vi "ClassPanel.vi"(8 "error in (no error)":errorcluster caption="entrée d'erreur (pas d'erreur)", 11 "AttoAMC.lvclass":refnum<class "AttoAMC.lvclass">) -> (0 "error out":errorcluster caption="sortie d'erreur", 3 "AttoAMC.lvclass Out":refnum<class "AttoAMC.lvclass">)   [LabVIEW 2019, in "AttoAMC.lvclass"]
uses:
  AttoAMC.lvclass
  C:/Programmes Labview/LabScanV1A/DevicesClass/BaseDevice/BaseDevice.lvclass
  AttoAMC.lvclass/AttoAMC.ctl
  BaseDevice/ClassQueueMess.ctl
  BaseDevice/Accessor/GetClassEvent.vi
panel:
  in  "FastScan":bool
  out "QuickPanRef":refnum<vi>
  in  "QuickPan":bool caption="MiseAJour"
  in  "AutoReset Ref":bool
  in  "Update Ref.":bool
  out "In Rng":bool
  in  "Target Rng":dbl=60.0 caption="Tgt. Rng.(nm)" min=1.0 step=1.0 format="%#.1f"
  out "Moving":bool
  out "ActVoltage":u32=60 caption="Act.Volt(mv)" min=1 step=1
  in  "Enable":bool
  out "Axis Model":string
  out "Valid Ref":bool
  out "BKD Lim":bool
  out "FWD Lim":bool
  in  "Axis":u8(ring) items=["1", "2", "3"]
  in  "MainProgQ":refnum<queue>
  in  "MainProgQEvent":refnum<user-event>
  out "RefPos":dbl=60.0 caption="Ref Pos(um)" min=0.1 step=0.1 format="%#.3f"
  in  "Freq.(Hz)":dbl
  in  "Ampl.(V)":dbl
  out "ActPos":dbl=60.0 caption="Actual Pos(um)" min=0.1 step=0.1 format="%#.3f"
  in  "Ctrl loop":bool
  in  "Read\nContin.":bool
  in  "Acq":bool
  in  "Stop":bool
  in  "Reset":bool caption="MiseAJour"
  in  "Target":dbl=60.0 caption="Target(um)" min=-25000.0 max=25000.0 step=0.001 format="%#.3f"
  out "Init Program":bool
  in  "Axis Name":string
  # "this MUST labeled with class name"
  # "this MUST be present and labeled \"Stop\" and \"Acq\""
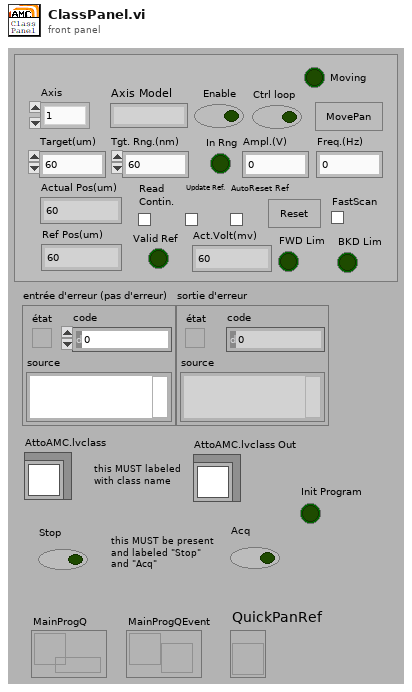
[diagram p1: front panel]
types:
  T1 = typedef "ClassQueueMess.ctl" = u16
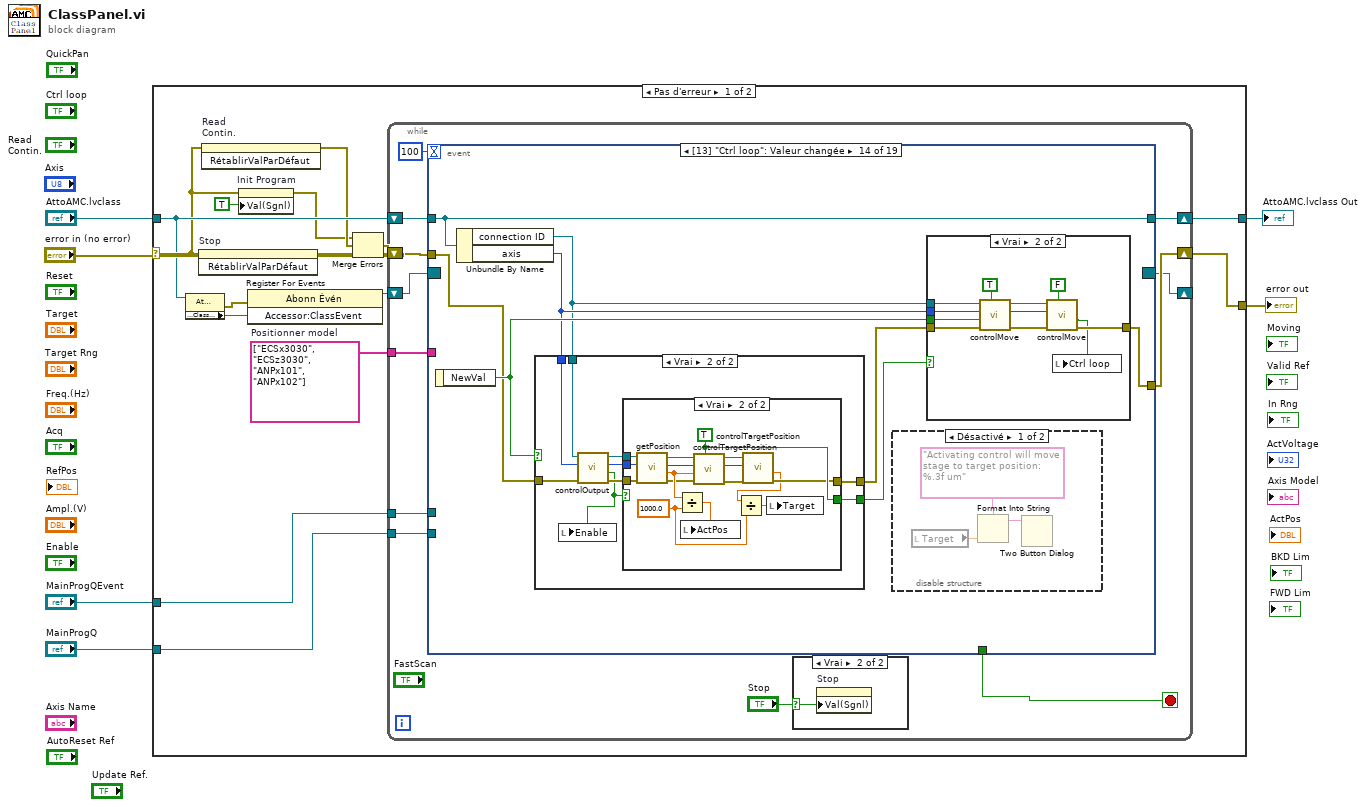
[diagram p0: block diagram]
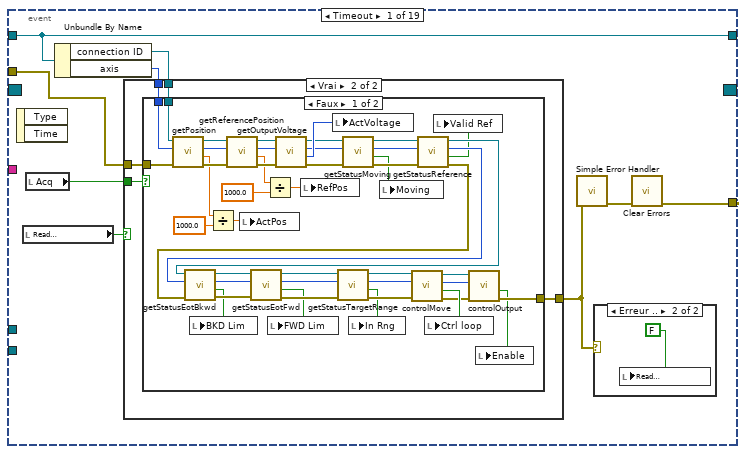
[diagram p3: hidden frame]
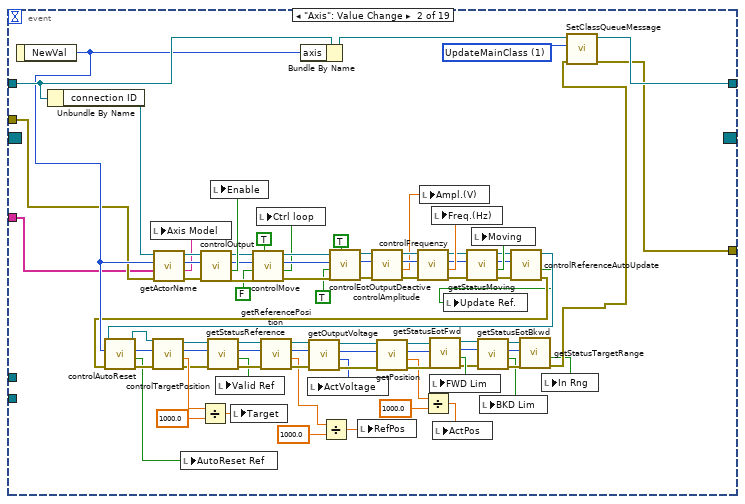
[diagram p7: hidden frame]
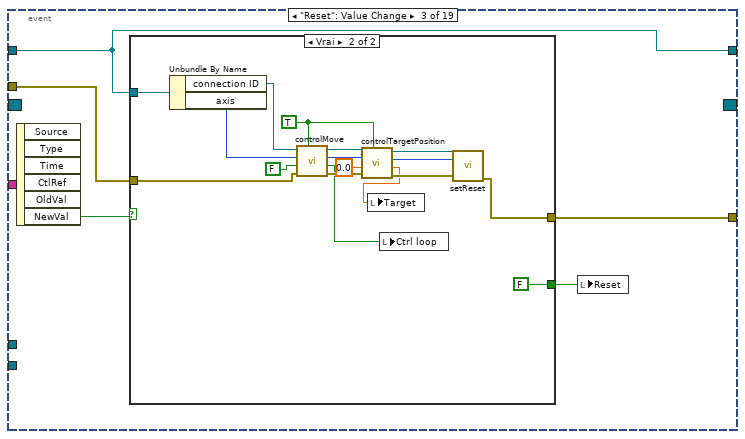
[diagram p8: hidden frame]
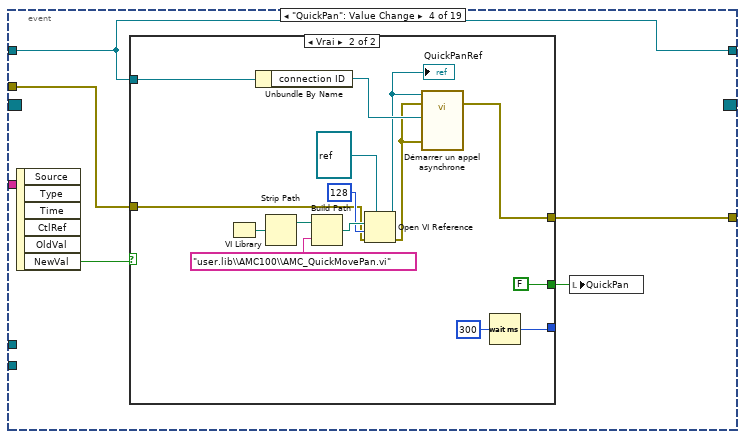
[diagram p10: hidden frame]
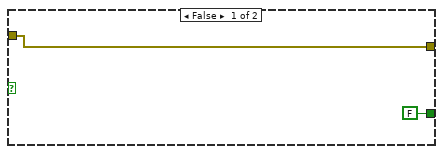
[diagram p11: hidden frame]
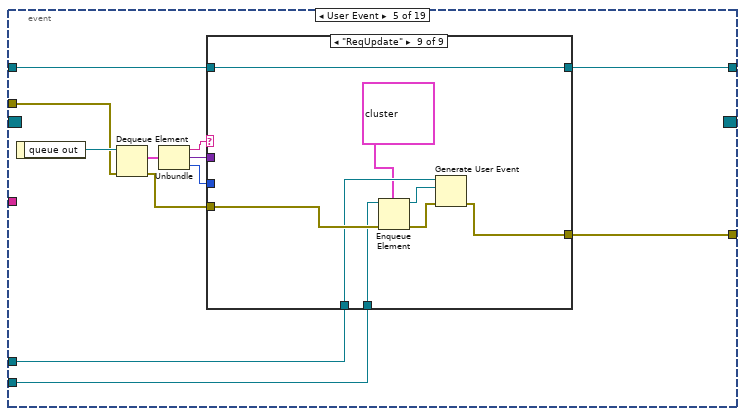
[diagram p12: hidden frame]
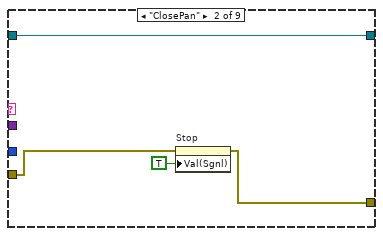
[diagram p14: hidden frame]
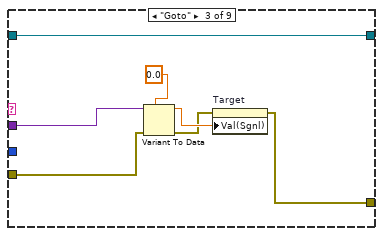
[diagram p15: hidden frame]
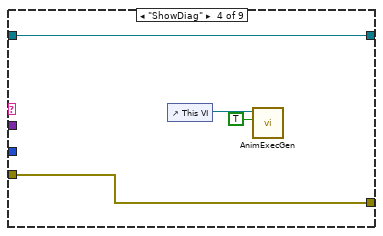
[diagram p16: hidden frame]
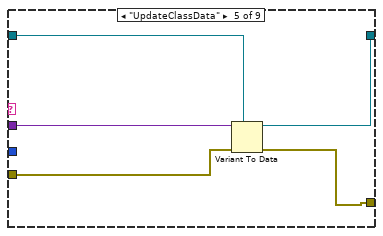
[diagram p17: hidden frame]
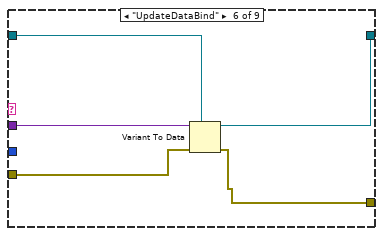
[diagram p18: hidden frame]
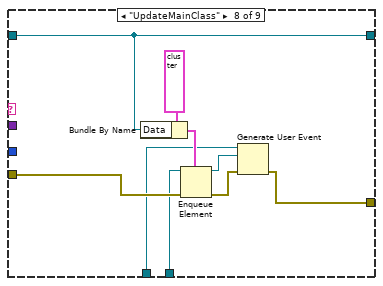
[diagram p20: hidden frame]
diagram:
  n1 = case shown="Pas d'erreur" "error in (no error)" {
    selector: "error in (no error)" -> [w8 w669]
    tunnel: [w21 w669] -> w5
    tunnel: "AttoAMC.lvclass" -> [w16 w668]
    tunnel: [w20 w668] -> w3
    tunnel: "MainProgQEvent" -> [w14 _]
    tunnel: "MainProgQ" -> [w13 _]
    frame No Error {
      w10 = string[] ["ECSx3030", "ECSz3030", "ANPx101", "ANPx102"]  # Positionner model
      n2 = property class="AttoAMC.lvclass"(reference=w16) -> (error out=w18:errorcluster, "Accessor:ClassEvent"=w17:refnum<user-event>)  [unwired: 1 in, 1 out]
      n3 = invoke on="Stop" class="Bool (strict)" method="RétablirValParDéfaut"(error in=w8) -> (error out=w19:errorcluster)  [unwired: 2 in, 2 out]
      n4 = invoke on="Read\nContin." class="Bool (strict)" method="RétablirValParDéfaut"(error in=w8) -> (error out=w11:errorcluster)  [unwired: 2 in, 2 out]
      n5 = property on="Init Program" class="Bool (strict)"(error in=w8, "Val(Sgnl)"=TRUE ("Valeur (Signalisation)")) -> (error out=w7:errorcluster)  [unwired: 1 in, 1 out]
      n6 = register-events(error in=w18, w17) -> (reference out=w15:refnum<event-registration>)  [unwired: 1 in, 1 out]
      n7 = Merge Errors(w7, w11, w19) -> (w12:errorcluster)
      n8 = while {
        shift-right: [w31] -> w21
        shift-left: w12 -> [w32]
        shift-right: [w29] -> w20
        shift-left: w16 -> [w30]
        shift-right: [w27] -> _
        shift-left: w15 -> [w28]
        tunnel: w14 -> [w26]
        tunnel: w13 -> [w25]
        tunnel: w10 -> [w24]
        stop <- w22 stop-if-true
        n9 = event shown="[13] \"Ctrl loop\": Valeur changée" {
          selector: w28 -> [_ _ _ _ _ _ _ _ _ _ _ _ _ _ _ _ _ _ _]
          dyn-events: [_ _ _ _ _ _ _ _ _ _ _ _ _ _ _ _ _ _ _] -> w27
          timeout: 100 -> [_ _ _ _ _ _ _ _ _ _ _ _ _ _ _ _ _ _ _]
          tunnel: w32 -> [w40 w172 w182 w205 w230 w290 w302 w314 w326 w338 w349 w391 w403 w414 w470 w493 w517 w615 w619]
          tunnel: [w42 w173 w181 w204 w232 w288 w301 w315 w327 w336 w348 w389 w401 w418 w466 w492 w520 _ w618] -> w31
          tunnel: w30 -> [w41 w176 w183 w206 w236 w293 w305 w322 w334 w346 w352 w399 w411 w419 w469 w490 w511 _ w620]
          tunnel: [_ _ _ _ _ _ _ _ _ _ _ _ _ _ _ w491 _ _ _] -> w22
          tunnel: [w41 w179 w183 w206 w231 w293 w305 w322 w334 w346 w352 w399 w411 w419 w468 w490 w519 _ w620] -> w29
          tunnel: w26 -> [_ _ _ _ w228 _ _ _ _ _ _ _ _ _ _ _ _ _ _]
          tunnel: w25 -> [_ _ _ _ w227 _ _ _ _ _ _ _ _ _ _ _ _ _ _]
          tunnel: w24 -> [_ w171 _ _ _ _ _ _ _ _ _ _ _ _ _ _ w518 _ _]
          event Timeout {
            n10 = event-data() -> ()  [unwired: 1 in, 2 out]
            n11 = local read "Read\nContin."() -> (w36:bool)
            n12 = local read "Acq"() -> (w37:bool)
            n13 = Unbundle By Name(w41) -> ("connection ID"=w39:refnum<k5>, "axis"=w38:u8)
            n14 = case shown="Vrai" w36 {
              tunnel: w40 -> [w45 w50]
              tunnel: [w45 w49] -> w35
              tunnel: w39 -> [_ w48]
              tunnel: w38 -> [_ w47]
              tunnel: w37 -> [_ w46]
              frame False {
              }
              frame True {
                n15 = case shown="Faux" w46 {
                  tunnel: w50 -> [w74 w96]
                  tunnel: [w54 w96] -> w49
                  tunnel: w48 -> [w73 _]
                  tunnel: w47 -> [w72 _]
                  frame False {
                    n16 = call <userlib>:"getPosition.vi"("error in"=w74, "axis in"=w72, "connection ID"=w73) -> ("error out"=w85:errorcluster, "position out"=w60:dbl, "axis out"=w94:u8, "connection ID"=w95:refnum<k5>)  [unwired: 5 in]
                    n17 = Divide(x=w60, y=1000.0) -> (x/y=w59:dbl)
                    n18 = call <userlib>:"getReferencePosition.vi"("error in"=w85, "axis in"=w94, "connection ID"=w95) -> ("error out"=w75:errorcluster, "Reference position out"=w57:dbl, "axis out"=w76:u8, "connection ID"=w77:refnum<k5>)  [unwired: 5 in]
                    n19 = local write "ActPos"(w59) -> ()
                    n20 = Divide(x=w57, y=1000.0) -> (x/y=w56:dbl)
                    n21 = call <userlib>:"getOutputVoltage.vi"("error in"=w75, "axis in"=w76, "connection ID"=w77) -> ("error out"=w70:errorcluster, "Voltage (mv)"=w71:i64, "axis out"=w68:u8, "connection ID"=w69:refnum<k5>)  [unwired: 5 in]
                    n22 = local write "RefPos"(w56) -> ()
                    n23 = local write "ActVoltage"(w71) -> ()
                    n24 = call <userlib>:"getStatusMoving.vi"("error in"=w70, "axis in"=w68, "connection ID"=w69) -> ("error out"=w84:errorcluster, "status moving out"=w67:bool, "axis out"=w92:u8, "connection ID"=w93:refnum<k5>)  [unwired: 5 in]
                    n25 = local write "Moving"(w67) -> ()
                    n26 = call <userlib>:"getStatusReference.vi"("error in"=w84, "axis in"=w92, "connection ID"=w93) -> ("error out"=w83:errorcluster, "status reference out"=w66:bool, "axis out"=w90:u8, "connection ID"=w91:refnum<k5>)  [unwired: 5 in]
                    n27 = call <userlib>:"getStatusEotBkwd.vi"("error in"=w83, "axis in"=w90, "connection ID"=w91) -> ("error out"=w82:errorcluster, "Get Stus EOT BKWD out"=w65:bool, "axis out"=w88:u8, "connection ID"=w89:refnum<k5>)  [unwired: 5 in]
                    n28 = local write "BKD Lim"(w65) -> ()
                    n29 = call <userlib>:"getStatusEotFwd.vi"("error in"=w82, "axis in"=w88, "connection ID"=w89) -> ("error out"=w81:errorcluster, "Status EOT FWD out"=w64:bool, "axis out"=w86:u8, "connection ID"=w87:refnum<k5>)  [unwired: 5 in]
                    n30 = local write "FWD Lim"(w64) -> ()
                    n31 = call <userlib>:"getStatusTargetRange.vi"("error in"=w81, "axis in"=w86, "connection ID"=w87) -> ("error out"=w78:errorcluster, "Status Target Range out"=w63:bool, "axis out"=w79:u8, "connection ID"=w80:refnum<k5>)  [unwired: 5 in]
                    n32 = local write "In Rng"(w63) -> ()
                    n33 = call <userlib>:"controlMove.vi"("error in"=w78, "axis in"=w79, "connection ID"=w80) -> ("error out"=w55:errorcluster, "controll move out"=w62:bool, "axis out"=w52:u8, "connection ID"=w51:refnum<k5>)  [unwired: 5 in]
                    n34 = local write "Ctrl loop"(w62) -> ()
                    n35 = local write "Valid Ref"(w66) -> ()
                    n36 = call <userlib>:"controlOutput.vi"("error in"=w55, "axis in"=w52, "connection ID"=w51) -> ("error out"=w54:errorcluster, "enable output out"=w53:bool)  [unwired: 5 in, 2 out]
                    n37 = local write "Enable"(w53) -> ()
                  }
                  frame True {
                  }
                }
              }
            }
            n38 = call <vilib>:"Simple Error Handler.vi"("error in (no error)"=w35) -> ("error out"=w43:errorcluster)  [unwired: 4 in, 4 out]
            n39 = case shown="Erreur .." w35 {
              frame No Error {
              }
              frame Error {
                n40 = local write "Read\nContin."(FALSE ("cas vrai")) -> ()
              }
            }
            n41 = call <vilib>:"Clear Errors.vi"("error in (no error)"=w43) -> ("error out"=w42:errorcluster)  [unwired: 5 in, 1 out]
          }
          event "Axis": Value Change {
            w178 = T1 1 items=["UpdateClassData", "UpdateMainClass"] ("Menu déroulant")
            n42 = event-data() -> ("NewVal"=w175:u8)  [unwired: 1 in]
            n43 = Unbundle By Name(w176) -> ("connection ID"=w97:refnum<k5>)
            n44 = call <userlib>:"getActorName.vi"("error in"=w172, "Actor Names"=w171, "axis in"=w175, "connection ID"=w97) -> ("error out"=w150:errorcluster, "ActorName out"=w125:string, "axis out"=w148:u8, "connection ID"=w149:refnum<k5>)  [unwired: 4 in]
            n45 = local write "Axis Model"(w125) -> ()
            n46 = call <userlib>:"controlOutput.vi"("error in"=w150, "axis in"=w148, "connection ID"=w149) -> ("error out"=w160:errorcluster, "enable output out"=w161:bool, "axis out"=w158:u8, "connection ID"=w159:refnum<k5>)  [unwired: 5 in]
            n47 = local write "Enable"(w161) -> ()
            n48 = call <userlib>:"controlMove.vi"("Set"=TRUE, "error in"=w160, "control move in"=FALSE, "axis in"=w158, "connection ID"=w159) -> ("error out"=w155:errorcluster, "controll move out"=w153:bool, "axis out"=w157:u8, "connection ID"=w156:refnum<k5>)  [unwired: 3 in]
            n49 = local write "Ctrl loop"(w153) -> ()
            n50 = Bundle By Name(cluster=w176, "axis"=w175) -> (w177:refnum<class "AttoAMC.lvclass">)
            n51 = call <userlib>:"controlEotOutputDeactive.vi"("Set"=TRUE, "error in"=w155, "enable EOT in"=TRUE, "axis in"=w157, "connection ID"=w156) -> ("error out"=w163:errorcluster, "axis out"=w162:u8, "connection ID"=w164:refnum<k5>)  [unwired: 3 in, 1 out]
            n52 = call <userlib>:"controlAmplitude.vi"("error in"=w163, "axis in"=w162, "connection ID"=w164) -> ("error out"=w168:errorcluster, "amplitude [V] out"=w166:dbl, "axis out"=w170:u8, "connection ID"=w169:refnum<k5>)  [unwired: 5 in]
            n53 = call <userlib>:"controlFrequenzy.vi"("error in"=w168, "axis in"=w170, "connection ID"=w169) -> ("error out"=w147:errorcluster, "Frequenzy [Hz] out"=w167:dbl, "axis out"=w145:u8, "connection ID"=w146:refnum<k5>)  [unwired: 5 in]
            n54 = local write "Ampl.(V)"(w166) -> ()
            n55 = local write "Freq.(Hz)"(w167) -> ()
            n56 = call <userlib>:"getStatusMoving.vi"("error in"=w147, "axis in"=w145, "connection ID"=w146) -> ("error out"=w104:errorcluster, "status moving out"=w103:bool, "axis out"=w102:u8, "connection ID"=w101:refnum<k5>)  [unwired: 5 in]
            n57 = local write "Moving"(w103) -> ()
            n58 = call <userlib>:"controlReferenceAutoUpdate.vi"("error in"=w104, "axis in"=w102, "connection ID"=w101) -> ("error out"=w100:errorcluster, "ref auto up out"=w98:bool, "connection ID"=w99:refnum<k5>)  [unwired: 5 in, 1 out]
            n59 = call <userlib>:"controlAutoReset.vi"("error in"=w100, "axis in"=w175, "connection ID"=w99) -> ("error out"=w108:errorcluster, "auto reset out"=w105:bool, "axis out"=w107:u8, "connection ID"=w106:refnum<k5>)  [unwired: 5 in]
            n60 = call <userlib>:"controlTargetPosition.vi"("error in"=w108, "axis in"=w107, "connection ID"=w106) -> ("error out"=w143:errorcluster, "Target Position out"=w144:dbl, "axis out"=w141:u8, "connection ID"=w142:refnum<k5>)  [unwired: 5 in]
            n61 = local write "AutoReset Ref"(w105) -> ()
            n62 = Divide(x=w144, y=1000.0) -> (x/y=w116:dbl)
            n63 = call <userlib>:"getStatusReference.vi"("error in"=w143, "axis in"=w141, "connection ID"=w142) -> ("error out"=w140:errorcluster, "status reference out"=w138:bool, "axis out"=w137:u8, "connection ID"=w139:refnum<k5>)  [unwired: 5 in]
            n64 = local write "Valid Ref"(w138) -> ()
            n65 = local write "Target"(w116) -> ()
            n66 = call <userlib>:"getReferencePosition.vi"("error in"=w140, "axis in"=w137, "connection ID"=w139) -> ("error out"=w136:errorcluster, "Reference position out"=w113:dbl, "axis out"=w134:u8, "connection ID"=w135:refnum<k5>)  [unwired: 5 in]
            n67 = call <userlib>:"getOutputVoltage.vi"("error in"=w136, "axis in"=w134, "connection ID"=w135) -> ("error out"=w133:errorcluster, "Voltage (mv)"=w130:i64, "axis out"=w131:u8, "connection ID"=w132:refnum<k5>)  [unwired: 5 in]
            n68 = local write "ActVoltage"(w130) -> ()
            n69 = Divide(x=w113, y=1000.0) -> (x/y=w112:dbl)
            n70 = local write "RefPos"(w112) -> ()
            n71 = call <userlib>:"getPosition.vi"("error in"=w133, "axis in"=w131, "connection ID"=w132) -> ("error out"=w128:errorcluster, "position out"=w110:dbl, "axis out"=w127:u8, "connection ID"=w129:refnum<k5>)  [unwired: 5 in]
            n72 = Divide(x=w110, y=1000.0) -> (x/y=w109:dbl)
            n73 = call <userlib>:"getStatusEotFwd.vi"("error in"=w128, "axis in"=w127, "connection ID"=w129) -> ("error out"=w124:errorcluster, "Status EOT FWD out"=w126:bool, "axis out"=w121:u8, "connection ID"=w122:refnum<k5>)  [unwired: 5 in]
            n74 = local write "FWD Lim"(w126) -> ()
            n75 = local write "ActPos"(w109) -> ()
            n76 = local write "Update Ref."(w98) -> ()
            n77 = call <userlib>:"getStatusEotBkwd.vi"("error in"=w124, "axis in"=w121, "connection ID"=w122) -> ("error out"=w123:errorcluster, "Get Stus EOT BKWD out"=w118:bool, "axis out"=w120:u8, "connection ID"=w119:refnum<k5>)  [unwired: 5 in]
            n78 = local write "BKD Lim"(w118) -> ()
            n79 = call <userlib>:"getStatusTargetRange.vi"("error in"=w123, "axis in"=w120, "connection ID"=w119) -> ("error out"=w174:errorcluster, "Status Target Range out"=w117:bool)  [unwired: 5 in, 2 out]
            n80 = local write "In Rng"(w117) -> ()
            n81 = call-dynamic "SetClassQueueMessage.vi"("ErrorIn(No Error)"=w174, "Menu déroulant"=w178, "DefaultDev.lvclass"=w177) -> ("sortie d'erreur"=w173:errorcluster, "DefaultDev.lvclass Out"=w179:refnum<class "AttoAMC.lvclass">)  [unwired: 7 in]
          }
          event "Reset": Value Change {
            n82 = event-data() -> ("NewVal"=w184:bool)  [unwired: 1 in, 5 out]
            n83 = case shown="Vrai" w184 {
              tunnel: w183 -> [_ w202]
              tunnel: w182 -> [w185 w197]
              tunnel: [w185 w201] -> w181
              tunnel: [_ FALSE] -> w180
              frame False {
              }
              frame True {
                w192 = TRUE ("Set")
                n84 = Unbundle By Name(w202) -> ("connection ID"=w199:refnum<k5>, "axis"=w198:u8)
                n85 = call <userlib>:"controlMove.vi"("Set"=w192, "error in"=w197, "control move in"=FALSE, "axis in"=w198, "connection ID"=w199) -> ("error out"=w195:errorcluster, "controll move out"=w186:bool, "axis out"=w194:u8, "connection ID"=w193:refnum<k5>)  [unwired: 3 in]
                n86 = call <userlib>:"controlTargetPosition.vi"("Set"=w192, "error in"=w195, "Target Position in"=0.0, "axis in"=w194, "connection ID"=w193) -> ("error out"=w190:errorcluster, "Target Position out"=w187:dbl, "axis out"=w188:u8, "connection ID"=w189:refnum<k5>)  [unwired: 3 in]
                n87 = local write "Target"(w187) -> ()
                n88 = local write "Ctrl loop"(w186) -> ()
                n89 = call <userlib>:"setReset.vi"("error in"=w190, "axis in"=w188, "connection ID"=w189) -> ("error out"=w201:errorcluster)  [unwired: 6 in, 2 out]
              }
            }
            n90 = local write "Reset"(w180) -> ()
          }
          event "QuickPan": Value Change {
            n91 = event-data() -> ("NewVal"=w207:bool)  [unwired: 1 in, 5 out]
            n92 = case shown="Vrai" w207 {
              tunnel: w206 -> [_ w214]
              tunnel: w205 -> [w209 w212]
              tunnel: [w209 w213] -> w204
              tunnel: [FALSE FALSE] -> w203
              tunnel: [_ w211] -> _
              frame False {
              }
              frame True {
                n93 = VI Library() -> (path=w221:path)
                n94 = Unbundle By Name(w214) -> ("connection ID"=w223:refnum<k5>)
                n95 = Strip Path(path=w221) -> (stripped path=w220:path)  [unwired: 1 out]
                n96 = Build Path(base path=w220, name or relative path="user.lib\\AMC100\\AMC_QuickMovePan.vi" ("nom ou chemin relatif")) -> (appended path=w219:path)
                n97 = Open VI Reference(type specifier VI Refnum (for type only)=refnum<vi> refnum ("spécificateur de type du refnum de VI (pour type seulement)"), vi path=w219, options=128, error in (no error)=w212) -> (vi reference=w216:refnum<vi>, error out=w217:errorcluster)  [unwired: 2 in]
                "QuickPanRef" <- w216
                n98 = call-by-ref "Démarrer un appel asynchrone"(reference=w216, error in=w217, 8:"error in (no error)"=w217, "ConnID"=w223) -> (error out=w213:errorcluster)  [unwired: 9 in, 2 out]
                n99 = Wait (ms)(milliseconds to wait=u32 300 ("attente (ms)")) -> (millisecond timer value=w211:u32)
              }
            }
            n100 = local write "QuickPan"(w203) -> ()
          }
          event User Event {
            n101 = event-data() -> ("queue out"=w234:refnum<queue>)  [unwired: 1 in]
            n102 = Dequeue Element(queue=w234, error in (no error)=w230) -> (element=w235:cluster{"Message":string, "Data":variant, i32}, error out=w229:errorcluster)  [unwired: 1 in, 2 out]
            n103 = Unbundle(w235) -> ("Message"=w226:string, "Data"=w233:variant, w225:i32)
            n104 = case shown="\"ReqUpdate\"" w226 {
              tunnel: w229 -> [w238 w241 w244 w253 w255 w260 w264 w269 w279]
              tunnel: w233 -> [_ _ w248 _ w258 w263 _ _ _]
              tunnel: w236 -> [w237 w242 w249 w252 w257 w262 w265 w270 w280]
              tunnel: [w237 w242 w249 w252 w256 w261 w265 w270 w280] -> w231
              tunnel: [w238 w240 w243 w253 w254 w259 w264 w266 w276] -> w232
              tunnel: w225 -> [_ _ _ _ _ _ _ _ _]
              tunnel: w228 -> [_ _ _ _ _ _ _ w268 w278]
              tunnel: w227 -> [_ _ _ _ _ _ _ w267 w277]
              frame Default {
              }
              frame "ClosePan" {
                n105 = property on="Stop" class="Bool (strict)"(error in=w241, "Val(Sgnl)"=TRUE ("Valeur (Signalisation)")) -> (error out=w240:errorcluster)  [unwired: 1 in, 1 out]
              }
              frame "Goto" {
                n106 = Variant To Data(error in=w244, type=0.0, Variant=w248) -> (data=w246:dbl, error out=w245:errorcluster)
                n107 = property on="Target" class="NumNb (strict)"(error in=w245, "Val(Sgnl)"=w246) -> (error out=w243:errorcluster)  [unwired: 1 in, 1 out]
              }
              frame "ShowDiag" {
                n108 = control-ref of="This VI"() -> (w251:refnum<vi>)
                n109 = call <userlib>:"AnimExecGen.vi"("Animer l'exécution ?"=TRUE, "ViRef"=w251) -> ()  [unwired: 9 in, 1 out]
              }
              frame "UpdateClassData" {
                n110 = Variant To Data(error in=w255, type=w257, Variant=w258) -> (data=w256:refnum<class "AttoAMC.lvclass">, error out=w254:errorcluster)
              }
              frame "UpdateDataBind" {
                n111 = Variant To Data(error in=w260, type=w262, Variant=w263) -> (data=w261:refnum<class "AttoAMC.lvclass">, error out=w259:errorcluster)
              }
              frame "MeasDone" {
              }
              frame "UpdateMainClass" {
                n112 = Bundle By Name(cluster=cluster{"Message":string, "Data":variant, i32} {"Message"="", "Data"=variant, 0} ("élément"), "Data"=w270) -> (w271:cluster{"Message":string, "Data":variant, i32})
                n113 = Enqueue Element(queue=w267, element=w271, error in (no error)=w269) -> (queue out=w274:refnum<queue>, error out=w273:errorcluster)  [unwired: 1 in, 1 out]
                n114 = Generate User Event(user event=w268, event data cluster=w274, error in=w273) -> (error out=w266:errorcluster)  [unwired: 1 in, 1 out]
              }
              frame "ReqUpdate" {
                n115 = Enqueue Element(queue=w277, element=cluster{"Message":string, "Data":variant, i32} {"Message"="ReqUpdate", "Data"=variant, 0} ("élément"), error in (no error)=w279) -> (queue out=w282:refnum<queue>, error out=w281:errorcluster)  [unwired: 1 in, 1 out]
                n116 = Generate User Event(user event=w278, event data cluster=w282, error in=w281) -> (error out=w276:errorcluster)  [unwired: 1 in, 1 out]
              }
            }
          }
          event "Target": Value Change {
            n117 = event-data() -> ("NewVal"=w289:dbl)  [unwired: 1 in]
            n118 = Unbundle By Name(w293) -> ("connection ID"=w292:refnum<k5>, "axis"=w291:u8)
            n119 = Multiply(x=w289, y=1000.0) -> (x*y=w287:dbl)
            n120 = call <userlib>:"controlTargetPosition.vi"("Set"=TRUE, "error in"=w290, "Target Position in"=w287, "axis in"=w291, "connection ID"=w292) -> ("error out"=w295:errorcluster, "axis out"=w296:u8, "connection ID"=w297:refnum<k5>)  [unwired: 3 in, 1 out]
            n121 = call <userlib>:"controlTargetPosition.vi"("Set"=FALSE, "error in"=w295, "axis in"=w296, "connection ID"=w297) -> ("error out"=w288:errorcluster, "Target Position out"=w284:dbl)  [unwired: 4 in, 2 out]
            n122 = Divide(x=w284, y=1000.0) -> (x/y=w283:dbl)
            n123 = local write "Target"(w283) -> ()
          }
          event "Target Rng": Value Change {
            n124 = event-data() -> ("NewVal"=w300:dbl)  [unwired: 1 in]
            n125 = Unbundle By Name(w305) -> ("connection ID"=w304:refnum<k5>, "axis"=w303:u8)
            n126 = call <userlib>:"controlTargetRange.vi"("Set"=TRUE, "error in"=w302, "Target Range in"=w300, "axis in"=w303, "connection ID"=w304) -> ("error out"=w307:errorcluster, "axis out"=w308:u8, "connection ID"=w309:refnum<k5>)  [unwired: 3 in, 1 out]
            n127 = call <userlib>:"controlTargetRange.vi"("Set"=FALSE, "error in"=w307, "axis in"=w308, "connection ID"=w309) -> ("error out"=w301:errorcluster, "Target Range out"=w299:dbl)  [unwired: 4 in, 2 out]
            n128 = local write "Target Rng"(w299) -> ()
          }
          event "Ampl.(V)": Value Change {
            n129 = event-data() -> ("NewVal"=w311:dbl)  [unwired: 1 in]
            n130 = Unbundle By Name(w322) -> ("connection ID"=w313:refnum<k5>, "axis"=w312:u8)
            n131 = call <userlib>:"controlAmplitude.vi"("Set"=TRUE, "error in"=w314, "amplitude [V] in"=w311, "axis in"=w312, "connection ID"=w313) -> ("error out"=w317:errorcluster, "axis out"=w319:u8, "connection ID"=w320:refnum<k5>)  [unwired: 3 in, 1 out]
            n132 = call <userlib>:"controlAmplitude.vi"("Set"=FALSE, "error in"=w317, "axis in"=w319, "connection ID"=w320) -> ("error out"=w315:errorcluster, "amplitude [V] out"=w316:dbl)  [unwired: 4 in, 2 out]
            n133 = local write "Ampl.(V)"(w316) -> ()
          }
          event "Freq.(Hz)": Value Change {
            n134 = event-data() -> ("NewVal"=w323:dbl)  [unwired: 1 in]
            n135 = Unbundle By Name(w334) -> ("connection ID"=w325:refnum<k5>, "axis"=w324:u8)
            n136 = call <userlib>:"controlFrequenzy.vi"("Set"=TRUE, "error in"=w326, "Frequenzy [Hz] in"=w323, "axis in"=w324, "connection ID"=w325) -> ("error out"=w329:errorcluster, "axis out"=w331:u8, "connection ID"=w332:refnum<k5>)  [unwired: 3 in, 1 out]
            n137 = call <userlib>:"controlFrequenzy.vi"("Set"=FALSE, "error in"=w329, "axis in"=w331, "connection ID"=w332) -> ("error out"=w327:errorcluster, "Frequenzy [Hz] out"=w328:dbl)  [unwired: 4 in, 2 out]
            n138 = local write "Freq.(Hz)"(w328) -> ()
          }
          event "Enable": Value Change {
            n139 = event-data() -> ("NewVal"=w337:bool)  [unwired: 1 in]
            n140 = Unbundle By Name(w346) -> ("connection ID"=w340:refnum<k5>, "axis"=w339:u8)
            n141 = call <userlib>:"controlOutput.vi"("Set"=TRUE, "error in"=w338, "enable output in"=w337, "axis in"=w339, "connection ID"=w340) -> ("error out"=w341:errorcluster, "axis out"=w342:u8, "connection ID"=w343:refnum<k5>)  [unwired: 3 in, 1 out]
            n142 = call <userlib>:"controlOutput.vi"("Set"=FALSE, "error in"=w341, "axis in"=w342, "connection ID"=w343) -> ("error out"=w336:errorcluster, "enable output out"=w335:bool)  [unwired: 4 in, 2 out]
            n143 = local write "Enable"(w335) -> ()
          }
          event "Enable": Shortcut Menu Selection (User) {
            n144 = event-data() -> ("ItemTag"=w347:string)  [unwired: 1 in, 3 out]
            n145 = Unbundle By Name(w352) -> ("connection ID"=w351:refnum<k5>, "axis"=w350:u8)
            n146 = case shown="\"Faux\", Par défaut" w347 {
              tunnel: w351 -> [_ w358 w375]
              tunnel: w350 -> [_ _ _]
              tunnel: w349 -> [w353 w357 w374]
              tunnel: [w353 w356 w373] -> w348
              frame "Faux", Default {
              }
              frame "EnableAll" {
                n147 = for {
                  N: 3 -> [_]
                  tunnel: w358 -> [w365]
                  tunnel: [w362] -> w355
                  shift-right: [w363] -> w356
                  shift-left: w357 -> [w364]
                  i -> [w360]
                  n148 = Increment(x=w360) -> (x+1=w361:i32)
                  n149 = call <userlib>:"controlOutput.vi"("Set"=TRUE, "error in"=w364, "enable output in"=TRUE, "axis in"=w361, "connection ID"=w365) -> ("error out"=w366:errorcluster, "axis out"=w367:u8, "connection ID"=w368:refnum<k5>)  [unwired: 3 in, 1 out]
                  n150 = call <userlib>:"controlOutput.vi"("Set"=FALSE, "error in"=w366, "axis in"=w367, "connection ID"=w368) -> ("error out"=w363:errorcluster, "enable output out"=w362:bool)  [unwired: 4 in, 2 out]
                }
                n151 = local write "Enable"(w355) -> ()
              }
              frame "DisableAll" {
                n152 = for {
                  N: 3 -> [_]
                  tunnel: w375 -> [w382]
                  tunnel: [w379] -> w372
                  shift-right: [w380] -> w373
                  shift-left: w374 -> [w381]
                  i -> [w377]
                  n153 = Increment(x=w377) -> (x+1=w378:i32)
                  n154 = call <userlib>:"controlOutput.vi"("Set"=TRUE, "error in"=w381, "enable output in"=FALSE, "axis in"=w378, "connection ID"=w382) -> ("error out"=w383:errorcluster, "axis out"=w384:u8, "connection ID"=w385:refnum<k5>)  [unwired: 3 in, 1 out]
                  n155 = call <userlib>:"controlOutput.vi"("Set"=FALSE, "error in"=w383, "axis in"=w384, "connection ID"=w385) -> ("error out"=w380:errorcluster, "enable output out"=w379:bool)  [unwired: 4 in, 2 out]
                }
                n156 = local write "Enable"(w372) -> ()
              }
            }
          }
          event "AutoReset Ref": Value Change {
            n157 = event-data() -> ("NewVal"=w390:bool)  [unwired: 1 in]
            n158 = Unbundle By Name(w399) -> ("connection ID"=w393:refnum<k5>, "axis"=w392:u8)
            n159 = call <userlib>:"controlAutoReset.vi"("Set"=TRUE, "error in"=w391, "auto reset in"=w390, "axis in"=w392, "connection ID"=w393) -> ("error out"=w394:errorcluster, "axis out"=w395:u8, "connection ID"=w396:refnum<k5>)  [unwired: 3 in, 1 out]
            n160 = call <userlib>:"controlAutoReset.vi"("Set"=FALSE, "error in"=w394, "axis in"=w395, "connection ID"=w396) -> ("error out"=w389:errorcluster, "auto reset out"=w388:bool)  [unwired: 4 in, 2 out]
            n161 = local write "AutoReset Ref"(w388) -> ()
          }
          event "Update Ref.": Value Change {
            n162 = event-data() -> ("NewVal"=w402:bool)  [unwired: 1 in]
            n163 = Unbundle By Name(w411) -> ("connection ID"=w405:refnum<k5>, "axis"=w404:u8)
            n164 = call <userlib>:"controlReferenceAutoUpdate.vi"("Set"=TRUE, "error in"=w403, "ref auto up in"=w402, "axis in"=w404, "connection ID"=w405) -> ("error out"=w406:errorcluster, "axis out"=w407:u8, "connection ID"=w408:refnum<k5>)  [unwired: 3 in, 1 out]
            n165 = call <userlib>:"controlReferenceAutoUpdate.vi"("Set"=FALSE, "error in"=w406, "axis in"=w407, "connection ID"=w408) -> ("error out"=w401:errorcluster, "ref auto up out"=w400:bool)  [unwired: 4 in, 2 out]
            n166 = local write "Update Ref."(w400) -> ()
          }
          event "Ctrl loop": Value Change {
            n167 = event-data() -> ("NewVal"=w417:bool)  [unwired: 1 in]
            n168 = Unbundle By Name(w419) -> ("connection ID"=w413:refnum<k5>, "axis"=w415:u8)
            n169 = case shown="Vrai" w417 {
              tunnel: [TRUE ("T button?") w426] -> w416
              tunnel: w415 -> [_ w433]
              tunnel: w414 -> [w423 w432]
              tunnel: w413 -> [_ w431]
              tunnel: [w423 w425] -> w412
              frame False {
              }
              frame True {
                n170 = call <userlib>:"controlOutput.vi"("error in"=w432, "axis in"=w433, "connection ID"=w431) -> ("error out"=w430:errorcluster, "enable output out"=w427:bool, "axis out"=w428:u8, "connection ID"=w429:refnum<k5>)  [unwired: 5 in]
                n171 = local write "Enable"(w427) -> ()
                n172 = case shown="Vrai" w427 {
                  tunnel: w430 -> [w434 w452]
                  tunnel: w429 -> [_ w451]
                  tunnel: w428 -> [_ w450]
                  tunnel: [FALSE w448] -> w426
                  tunnel: [w434 w438] -> w425
                  frame False {
                    n173 = One Button Dialog(message="Axis is not Enable!") -> ()  [unwired: 1 in, 1 out]
                  }
                  frame True {
                    w448 = TRUE ("Set")
                    w442 = 1000.0 ("y")
                    n174 = call <userlib>:"getPosition.vi"("error in"=w452, "axis in"=w450, "connection ID"=w451) -> ("error out"=w444:errorcluster, "position out"=w447:dbl, "axis out"=w445:u8, "connection ID"=w446:refnum<k5>)  [unwired: 5 in]
                    n175 = Divide(x=w447, y=w442) -> (x/y=w449:dbl)
                    n176 = local write "ActPos"(w449) -> ()
                    n177 = call <userlib>:"controlTargetPosition.vi"("Set"=w448, "error in"=w444, "Target Position in"=w447, "axis in"=w445, "connection ID"=w446) -> ("error out"=w441:errorcluster, "axis out"=w440:u8, "connection ID"=w439:refnum<k5>)  [unwired: 3 in, 1 out]
                    n178 = call <userlib>:"controlTargetPosition.vi"("error in"=w441, "axis in"=w440, "connection ID"=w439) -> ("error out"=w438:errorcluster, "Target Position out"=w437:dbl)  [unwired: 5 in, 2 out]
                    n179 = Divide(x=w437, y=w442) -> (x/y=w443:dbl)
                    n180 = local write "Target"(w443) -> ()
                  }
                }
              }
            }
            n181 = disable-structure shown="Désactivé" {
              frame Disabled {
                n182 = local read "Target"() -> (w421:dbl)
                n183 = Format Into String(format string="Activating control will move stage to target position: %.3f um" ("message"), w421) -> (resulting string=w422:string)  [unwired: 2 in, 1 out]
                n184 = Two Button Dialog(message=w422) -> ()  [unwired: 2 in, 1 out]
              }
              frame Enabled {
              }
            }
            n185 = case shown="Vrai" w416 {
              tunnel: w412 -> [w453 w460]
              tunnel: w417 -> [_ w459]
              tunnel: w415 -> [_ w458]
              tunnel: w413 -> [_ w457]
              tunnel: [w453 w456] -> w418
              frame False {
                n186 = local write "Ctrl loop"(FALSE ("Control loop")) -> ()
              }
              frame True {
                n187 = call <userlib>:"controlMove.vi"("Set"=TRUE, "error in"=w460, "control move in"=w459, "axis in"=w458, "connection ID"=w457) -> ("error out"=w461:errorcluster, "axis out"=w462:u8, "connection ID"=w465:refnum<k5>)  [unwired: 3 in, 1 out]
                n188 = call <userlib>:"controlMove.vi"("Set"=FALSE, "error in"=w461, "axis in"=w462, "connection ID"=w465) -> ("error out"=w456:errorcluster, "controll move out"=w455:bool)  [unwired: 4 in, 2 out]
                n189 = local write "Ctrl loop"(w455) -> ()
              }
            }
          }
          event "Axis Name": Shortcut Menu Selection (User) {
            n190 = event-data() -> ("ItemTag"=w467:string)  [unwired: 1 in]
            n191 = case shown="\"ChangeName\"" w467 {
              tunnel: w470 -> [w471 w480]
              tunnel: w469 -> [w472 w478]
              tunnel: [w472 w475] -> w468
              tunnel: [w471 w473] -> w466
              frame Default {
              }
              frame "ChangeName" {
                n192 = call "SaveAxisName"("Enable"=TRUE, "error in (no error)"=w480) -> ("Name"=w477:string, "Save"=w476:bool, "error out"=w474:errorcluster)  [unwired: 15 in]
                n193 = case shown="Vrai" w476 {
                  tunnel: w478 -> [w482 w489]
                  tunnel: w477 -> [_ w483]
                  tunnel: [w482 w487] -> w475
                  tunnel: w474 -> [w481 w486]
                  tunnel: [w481 w484] -> w473
                  frame False {
                  }
                  frame True {
                    w485 = T1 1 items=["UpdateClassData", "UpdateMainClass"] ("Menu déroulant")
                    n194 = Bundle By Name(cluster=w489, "AxisName"=w483) -> (w488:refnum<class "AttoAMC.lvclass">)
                    n195 = local write "Axis Name"(w483) -> ()
                    n196 = call-dynamic "SetClassQueueMessage.vi"("ErrorIn(No Error)"=w486, "Menu déroulant"=w485, "DefaultDev.lvclass"=w488) -> ("sortie d'erreur"=w484:errorcluster, "DefaultDev.lvclass Out"=w487:refnum<class "AttoAMC.lvclass">)  [unwired: 7 in]
                  }
                }
              }
            }
          }
          event "Stop": Value Change {
            n197 = event-data() -> ("NewVal"=w491:bool)  [unwired: 1 in, 5 out]
            n198 = case shown="Vrai" w491 {
              tunnel: w490 -> [_ w503]
              tunnel: w493 -> [w494 w497]
              tunnel: [w494 w496] -> w492
              frame False {
              }
              frame True {
                n199 = local read "QuickPanRef"() -> (w498:refnum<vi>)
                n200 = Unbundle By Name(w503) -> ("connection ID"=w500:refnum<k5>)
                n201 = Not A Number/Path/Refnum?(number/path/refnum=w498) -> (NaN/Path/Refnum?=w499:bool)
                n202 = case shown="Faux" w499 {
                  tunnel: w498 -> [w508 _]
                  tunnel: w497 -> [w507 w509]
                  tunnel: [w505 w509] -> w495
                  frame False {
                    n203 = invoke class="Type d'interface de VI 0" method="ValCmde.Déf"(reference=w508, error in=w507, "Control Name"="Quit" ("Nom de la commande"), "Value"=TRUE) -> (error out=w505:errorcluster)  [unwired: 1 in, 4 out]
                  }
                  frame True {
                  }
                }
                n204 = call <userlib>:"AMC_OpenCloseConn.vi"("Open"=FALSE, "error in"=w497, "ConnID"=w500) -> ("error out"=w502:errorcluster)  [unwired: 7 in, 1 out]
                n205 = Merge Errors(w502, w495) -> (w496:errorcluster)
              }
            }
          }
          event "Init Program": Value Change {
            n206 = event-data() -> ()  [unwired: 1 in, 1 out]
            n207 = Unbundle By Name(w511) -> ("axis"=w514:u8, "AxisName"=w513:string)
            n208 = property class="AttoAMC.lvclass"(reference=w511) -> ("Accessor:VisaRes"=w510:refnum<visa-resource-name>)  [unwired: 1 in, 2 out]
            n209 = call <userlib>:"AMC_OpenCloseConn.vi"("Open"=TRUE, "error in"=w517, "deviceAddress"=w510) -> ("error out"=w512:errorcluster, "connection ID"=w516:refnum<k5>)  [unwired: 7 in]
            n210 = case shown="Pas d'erreur" w512 {
              selector: w512 -> [w521 w612]
              tunnel: [w579 w608] -> w520
              tunnel: w511 -> [w602 w613]
              tunnel: [w604 w613] -> w519
              tunnel: w518 -> [w575 _]
              tunnel: w516 -> [w531 _]
              tunnel: w514 -> [w533 _]
              tunnel: w513 -> [w532 _]
              frame No Error {
                w523 = 1000.0 ("y")
                w606 = T1 1 items=["UpdateClassData", "UpdateMainClass"] ("Menu déroulant")
                n211 = local write "Axis"(w533) -> ()
                n212 = call <userlib>:"getActorName.vi"("error in"=w521, "Actor Names"=w575, "axis in"=w533, "connection ID"=w531) -> ("error out"=w582:errorcluster, "ActorName out"=w558:string, "axis out"=w580:u8, "connection ID"=w581:refnum<k5>)  [unwired: 4 in]
                n213 = local write "Axis Model"(w558) -> ()
                n214 = local write "Axis Name"(w532) -> ()
                n215 = call <userlib>:"controlOutput.vi"("error in"=w582, "axis in"=w580, "connection ID"=w581) -> ("error out"=w591:errorcluster, "enable output out"=w592:bool, "axis out"=w589:u8, "connection ID"=w590:refnum<k5>)  [unwired: 5 in]
                n216 = local write "Enable"(w592) -> ()
                n217 = call <userlib>:"controlMove.vi"("Set"=FALSE, "error in"=w591, "axis in"=w589, "connection ID"=w590) -> ("error out"=w586:errorcluster, "controll move out"=w584:bool, "axis out"=w588:u8, "connection ID"=w587:refnum<k5>)  [unwired: 4 in]
                n218 = local write "Ctrl loop"(w584) -> ()
                n219 = Bundle By Name(cluster=w602, "connection ID"=w531) -> (w605:refnum<class "AttoAMC.lvclass">)
                n220 = call <userlib>:"controlEotOutputDeactive.vi"("Set"=TRUE, "error in"=w586, "enable EOT in"=TRUE, "axis in"=w588, "connection ID"=w587) -> ("error out"=w594:errorcluster, "axis out"=w593:u8, "connection ID"=w595:refnum<k5>)  [unwired: 3 in, 1 out]
                n221 = call <userlib>:"controlAmplitude.vi"("error in"=w594, "axis in"=w593, "connection ID"=w595) -> ("error out"=w599:errorcluster, "amplitude [V] out"=w597:dbl, "axis out"=w601:u8, "connection ID"=w600:refnum<k5>)  [unwired: 5 in]
                n222 = call <userlib>:"controlFrequenzy.vi"("error in"=w599, "axis in"=w601, "connection ID"=w600) -> ("error out"=w578:errorcluster, "Frequenzy [Hz] out"=w598:dbl, "axis out"=w576:u8, "connection ID"=w577:refnum<k5>)  [unwired: 5 in]
                n223 = local write "Ampl.(V)"(w597) -> ()
                n224 = local write "Freq.(Hz)"(w598) -> ()
                n225 = call <userlib>:"getStatusMoving.vi"("error in"=w578, "axis in"=w576, "connection ID"=w577) -> ("error out"=w539:errorcluster, "status moving out"=w538:bool, "axis out"=w537:u8, "connection ID"=w536:refnum<k5>)  [unwired: 5 in]
                n226 = local write "Moving"(w538) -> ()
                n227 = call <userlib>:"controlReferenceAutoUpdate.vi"("error in"=w539, "axis in"=w537, "connection ID"=w536) -> ("error out"=w535:errorcluster, "ref auto up out"=w534:bool)  [unwired: 5 in, 2 out]
                n228 = call <userlib>:"controlAutoReset.vi"("error in"=w535, "axis in"=w533, "connection ID"=w531) -> ("error out"=w543:errorcluster, "auto reset out"=w540:bool, "axis out"=w542:u8, "connection ID"=w541:refnum<k5>)  [unwired: 5 in]
                n229 = call <userlib>:"controlTargetPosition.vi"("error in"=w543, "axis in"=w542, "connection ID"=w541) -> ("error out"=w530:errorcluster, "Target Position out"=w529:dbl, "axis out"=w528:u8, "connection ID"=w525:refnum<k5>)  [unwired: 5 in]
                n230 = local write "AutoReset Ref"(w540) -> ()
                n231 = call <userlib>:"controlTargetRange.vi"("error in"=w530, "axis in"=w528, "connection ID"=w525) -> ("error out"=w527:errorcluster, "Target Range out"=w522:dbl, "axis out"=w526:u8, "connection ID"=w524:refnum<k5>)  [unwired: 5 in]
                n232 = Divide(x=w529, y=w523) -> (x/y=w549:dbl)
                n233 = local write "Target"(w549) -> ()
                n234 = call <userlib>:"getStatusReference.vi"("error in"=w527, "axis in"=w526, "connection ID"=w524) -> ("error out"=w574:errorcluster, "status reference out"=w572:bool, "axis out"=w571:u8, "connection ID"=w573:refnum<k5>)  [unwired: 5 in]
                n235 = local write "Target Rng"(w522) -> ()
                n236 = local write "Valid Ref"(w572) -> ()
                n237 = call <userlib>:"getReferencePosition.vi"("error in"=w574, "axis in"=w571, "connection ID"=w573) -> ("error out"=w570:errorcluster, "Reference position out"=w548:dbl, "axis out"=w568:u8, "connection ID"=w569:refnum<k5>)  [unwired: 5 in]
                n238 = Divide(x=w548, y=w523) -> (x/y=w547:dbl)
                n239 = call <userlib>:"getOutputVoltage.vi"("error in"=w570, "axis in"=w568, "connection ID"=w569) -> ("error out"=w567:errorcluster, "Voltage (mv)"=w564:i64, "axis out"=w565:u8, "connection ID"=w566:refnum<k5>)  [unwired: 5 in]
                n240 = local write "ActVoltage"(w564) -> ()
                n241 = local write "RefPos"(w547) -> ()
                n242 = call <userlib>:"getPosition.vi"("error in"=w567, "axis in"=w565, "connection ID"=w566) -> ("error out"=w562:errorcluster, "position out"=w545:dbl, "axis out"=w561:u8, "connection ID"=w563:refnum<k5>)  [unwired: 5 in]
                n243 = Divide(x=w545, y=1000.0) -> (x/y=w544:dbl)
                n244 = call <userlib>:"getStatusEotFwd.vi"("error in"=w562, "axis in"=w561, "connection ID"=w563) -> ("error out"=w557:errorcluster, "Status EOT FWD out"=w560:bool, "axis out"=w554:u8, "connection ID"=w555:refnum<k5>)  [unwired: 5 in]
                n245 = local write "FWD Lim"(w560) -> ()
                n246 = local write "ActPos"(w544) -> ()
                n247 = local write "Update Ref."(w534) -> ()
                n248 = call <userlib>:"getStatusEotBkwd.vi"("error in"=w557, "axis in"=w554, "connection ID"=w555) -> ("error out"=w556:errorcluster, "Get Stus EOT BKWD out"=w551:bool, "axis out"=w553:u8, "connection ID"=w552:refnum<k5>)  [unwired: 5 in]
                n249 = local write "BKD Lim"(w551) -> ()
                n250 = call-dynamic "SetClassQueueMessage.vi"("ErrorIn(No Error)"=w521, "Menu déroulant"=w606, "DefaultDev.lvclass"=w605) -> ("sortie d'erreur"=w603:errorcluster, "DefaultDev.lvclass Out"=w604:refnum<class "AttoAMC.lvclass">)  [unwired: 7 in]
                n251 = call <userlib>:"getStatusTargetRange.vi"("error in"=w556, "axis in"=w553, "connection ID"=w552) -> ("error out"=w559:errorcluster, "Status Target Range out"=w550:bool)  [unwired: 5 in, 2 out]
                n252 = local write "In Rng"(w550) -> ()
                n253 = Merge Errors(w603, w559) -> (w579:errorcluster)
                "Init Program" <- FALSE
              }
              frame Error {
                w610 = 1 items=["pas d'exception", "annuler l'erreur", "définir l'erreur"] ("[exception action] (none:0)")
                n254 = call <vilib>:"General Error Handler.vi"("error in (no error)"=w612, "[exception action] (none:0)"=w610, "[exception code]"=5000) -> ("error out"=w609:errorcluster)  [unwired: 8 in, 4 out]
                n255 = call <vilib>:"Clear Errors.vi"("error in (no error)"=w609) -> ("error out"=w608:errorcluster)  [unwired: 5 in, 1 out]
              }
            }
          }
          event "FWD Lim", "BKD Lim": Value Change {
            n256 = event-data() -> ("CtlRef"=w617:refnum<vi>, "NewVal"=w614:bool)  [unwired: 1 in, 4 out]
            n257 = property class="Bool (strict)"(reference=w617, error in=w615) -> ("Label.Text"=w616:string)  [unwired: 2 out]
            n258 = case shown="\"FWD Lim\"" w616 {
              tunnel: w614 -> [_ _ _]
              frame Default {
              }
              frame "BKD Lim" {
              }
              frame "FWD Lim" {
              }
            }
          }
          event "Moving": Value Change {
            n259 = event-data() -> ("NewVal"=w623:bool)  [unwired: 1 in]
            n260 = Unbundle By Name(w620) -> ("connection ID"=w622:refnum<k5>, "axis"=w621:u8)
            n261 = case shown="Vrai" w623 {
              tunnel: w619 -> [w624 w631]
              tunnel: [w624 w625] -> w618
              tunnel: w622 -> [_ w630]
              tunnel: w621 -> [_ w629]
              frame False {
              }
              frame True {
                n262 = while {
                  tunnel: w630 -> [w663]
                  tunnel: w629 -> [w662]
                  shift-right: [w646] -> w626
                  shift-left: w631 -> [w664]
                  tunnel: [w644] -> w628
                  tunnel: [w643] -> w627
                  stop <- w645 stop-if-true
                  n263 = Wait (ms)(milliseconds to wait=u32 50 ("attente (ms)")) -> ()  [unwired: 1 out]
                  n264 = call <userlib>:"getPosition.vi"("error in"=w664, "axis in"=w662, "connection ID"=w663) -> ("error out"=w653:errorcluster, "position out"=w656:dbl, "connection ID"=w654:refnum<k5>)  [unwired: 5 in, 1 out]
                  n265 = Divide(x=w656, y=1000.0) -> (x/y=w655:dbl)
                  n266 = call <userlib>:"getOutputVoltage.vi"("error in"=w653, "connection ID"=w654) -> ("error out"=w660:errorcluster, "Voltage (mv)"=w661:i64, "axis out"=w658:u8, "connection ID"=w659:refnum<k5>)  [unwired: 6 in]
                  n267 = local write "ActVoltage"(w661) -> ()
                  n268 = local write "ActPos"(w655) -> ()
                  n269 = call <userlib>:"getStatusMoving.vi"("error in"=w660, "axis in"=w658, "connection ID"=w659) -> ("error out"=w650:errorcluster, "status moving out"=w647:bool, "axis out"=w651:u8, "connection ID"=w652:refnum<k5>)  [unwired: 5 in]
                  n270 = call <userlib>:"getStatusEotBkwd.vi"("error in"=w650, "axis in"=w651, "connection ID"=w652) -> ("error out"=w665:errorcluster, "Get Stus EOT BKWD out"=w649:bool, "axis out"=w666:u8, "connection ID"=w667:refnum<k5>)  [unwired: 5 in]
                  n271 = local write "BKD Lim"(w649) -> ()
                  n272 = call <userlib>:"getStatusEotFwd.vi"("error in"=w665, "axis in"=w666, "connection ID"=w667) -> ("error out"=w646:errorcluster, "Status EOT FWD out"=w643:bool)  [unwired: 5 in, 2 out]
                  n273 = local write "FWD Lim"(w643) -> ()
                  n274 = local write "Moving"(w647) -> ()
                  n275 = Compound Arithmetic op=AND ("Opérateur arithmétique")(invert w643, invert w649) -> (w644:bool)
                  n276 = Compound Arithmetic op=AND ("Opérateur arithmétique")(w646, invert w647, w644) -> (w645:bool)
                }
                n277 = case shown="Vrai" w628 {
                  selector: w628 -> [_ w635]
                  tunnel: w627 -> [_ w636]
                  tunnel: w626 -> [w632 w634]
                  tunnel: [w632 w633] -> w625
                  frame False {
                  }
                  frame True {
                    n278 = case shown="Vrai" w636 {
                      tunnel: w635 -> [w639 w642]
                      tunnel: w634 -> [w638 w641]
                      tunnel: [w637 w640] -> w633
                      frame True {
                        n279 = property on="FWD Lim" class="Bool (strict)"(error in=w638, "Val(Sgnl)"=w639) -> (error out=w637:errorcluster)  [unwired: 1 in, 1 out]
                      }
                      frame False {
                        n280 = property on="BKD Lim" class="Bool (strict)"(error in=w641, "Val(Sgnl)"=w642) -> (error out=w640:errorcluster)  [unwired: 1 in, 1 out]
                      }
                    }
                  }
                }
              }
            }
          }
        }
        n281 = case shown="Vrai" "Stop" {
          selector: "Stop" -> [_ w34]
          frame False {
          }
          frame True {
            n282 = property on="Stop" class="Bool (strict)"("Val(Sgnl)"=w34) -> ()  [unwired: 2 in, 2 out]
          }
        }
      }
    }
    frame Error {
    }
  }
  "error out" <- w5
  "AttoAMC.lvclass Out" <- w3
